vi "TDTRX6-Start.vi"(4 "error in (no error)":errorcluster) -> (0 "error out":errorcluster)   [LabVIEW 2020]
doc: "Sends <B>Start</B> notifier to DAQ thread to begin measurement."
uses:
  TDT-Globals.vi
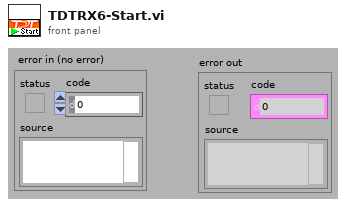
[diagram p1: front panel]
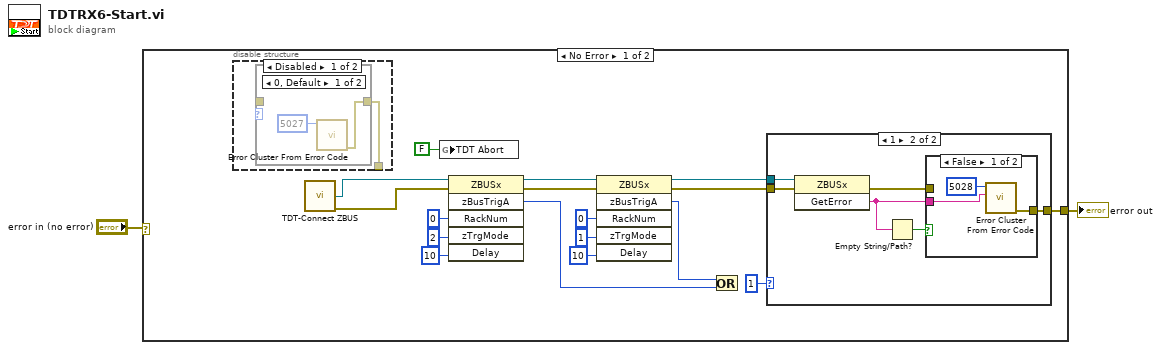
[diagram p0: block diagram]
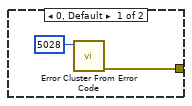
[diagram p4: hidden frame]
diagram:
  n1 = case shown="No Error" "error in (no error)" {
    selector: "error in (no error)" -> [_ w36]
    tunnel: [w9 w36] -> w1
    frame No Error {
      n2 = disable-structure shown="Disabled" {
        disable-tunnel: [w20 _] -> _
        frame Disabled {
          n3 = case shown="0, Default" {
            selector: _ -> [_ _]
            tunnel: _ -> [_ w23]
            tunnel: [w21 w23] -> w20
            frame 0, Default {
              n4 = call <vilib>:"Error Cluster From Error Code.vi"("error code (0)"=5027) -> ("error out"=w21:errorcluster)  [unwired: 8 in]
            }
            frame 1 {
            }
          }
        }
        frame Enabled {
        }
      }
      n5 = call "TDT-Connect ZBUS.vi"() -> ("ZBUSx"=w4:refnum<k7>, "error out"=w3:errorcluster)  [unwired: 14 in]
      n6 = global write "TDT-Globals.vi" "TDT Abort"(FALSE ("TDT Abort")) -> ()
      n7 = invoke class="ZBUSx" method="zBusTrigA"(reference=w4, error in=w3, "RackNum"=0, "zTrgMode"=2, "Delay"=10) -> (reference out=w13:refnum<k7>, error out=w12:errorcluster, "zBusTrigA"=w10:i32)  [unwired: 1 in, 3 out]
      n8 = invoke class="ZBUSx" method="zBusTrigA"(reference=w13, error in=w12, "RackNum"=0, "zTrgMode"=1, "Delay"=10) -> (reference out=w7:refnum<k7>, error out=w8:errorcluster, "zBusTrigA"=w11:i32)  [unwired: 1 in, 3 out]
      n9 = Or(x=w11, y=w10) -> ()  [unwired: 1 out]
      n10 = case shown="1" 1 {
        tunnel: [w24 w26] -> w9
        tunnel: w8 -> [_ w31]
        tunnel: w7 -> [_ w30]
        frame 0, Default {
          n11 = call <vilib>:"Error Cluster From Error Code.vi"("error code (0)"=5028) -> ("error out"=w24:errorcluster)  [unwired: 8 in]
        }
        frame 1 {
          n12 = invoke class="ZBUSx" method="GetError"(reference=w30, error in=w31) -> (error out=w29:errorcluster, "GetError"=w27:string)  [unwired: 1 in, 1 out]
          n13 = Empty String/Path?(string/path=w27) -> (empty?=w28:bool)
          n14 = case shown="False" w28 {
            tunnel: w29 -> [_ w35]
            tunnel: w27 -> [w33 _]
            tunnel: [w32 w35] -> w26
            frame False {
              n15 = call <vilib>:"Error Cluster From Error Code.vi"("error message (\"\")"=w33, "error code (0)"=5028) -> ("error out"=w32:errorcluster)  [unwired: 7 in]
            }
            frame True {
            }
          }
        }
      }
    }
    frame Error {
    }
  }
  "error out" <- w1
